vi "CLSUIP_SetNmdBundlerElement.vi"(8 "error in (no error)":errorcluster, 10 "Element Names":string[](array[string]), 11 "NmdBundler Ref":refnum<vi>) -> (0 "error out":errorcluster, 3 "NmdBundler Ref out":refnum<vi>)   [LabVIEW 2019, in "BlueBranch_CLSUIP.lvlib"]
uses:
  BlueBranch_CLSUIP.lvlib
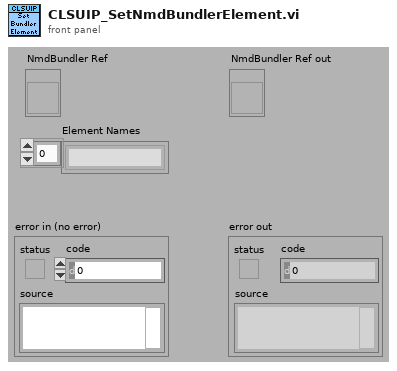
[diagram p1: front panel]
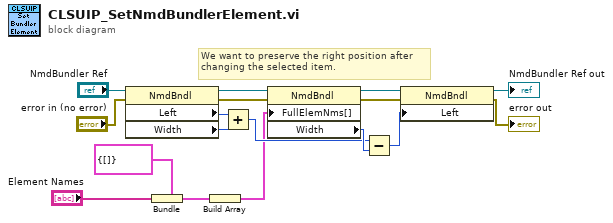
[diagram p0: block diagram]
diagram:
  # "We want to preserve the right position after\nchanging the selected item."
  n1 = property class="NmdBndl"(reference="NmdBundler Ref", error in="error in (no error)") -> (reference out=w13:refnum<vi>, error out=w12:errorcluster, "Left"=w15:i32, "Width"=w14:u32)
  n2 = Bundle(cluster=cluster{string[]} {[]}, "Element Names") -> (w2:cluster{string[]})
  n3 = Build Array(w2) -> (w1:cluster{string[]}[])
  n4 = Add(x=w15, y=w14) -> (x+y=w8:u32)
  n5 = property class="NmdBndl"(reference=w13, error in=w12, "FullElemNms[]"=w1) -> (reference out=w11:refnum<vi>, error out=w10:errorcluster, "Width"=w9:u32)
  n6 = Subtract(x=w8, y=w9) -> (x-y=w7:u32)
  n7 = property class="NmdBndl"(reference=w11, error in=w10, "Left"=w7) -> (reference out=→"NmdBundler Ref out":refnum<vi>, error out=→"error out":errorcluster)
